vi "INI Use Position Size.vi"(8 "error in":errorcluster, 11 "Editor Position in":refnum<class "Editor Position.lvclass">) -> (0 "error out":errorcluster, 3 "Editor Position out":refnum<class "Editor Position.lvclass">)   [LabVIEW 2021, in "Editor Position.lvclass"]
doc: "Tests the reading of the Use Position Size INI key."
uses:
  Editor Position.lvclass
  C:/Program Files/National Instruments/LabVIEW 2024/vi.lib/Astemes/LUnit/Test Case.lvclass
  <vilib>/Astemes/LUnit/Test Case.lvclass/Test Case.ctl
  <vilib>/Astemes/LUnit/Core/LUnit Test Case/Private/Append Pass Result.vi
  <vilib>/Astemes/LUnit/Core/LUnit Test Case/Private/Append Fail Result.vi
  <vilib>/Astemes/LUnit/Core/LUnit Test Case/Private/Run In UI.vi
  <vilib>/Utility/error.llb/Clear Errors.vi
  <resource>/dialog/lvconfig.llb/LV Config Write Boolean.vi
  <vilib>/LabVIEW Icon API/lv_icon/lv_icon.lvlib
  <vilib>/Astemes/LUnit/Test Case.lvclass
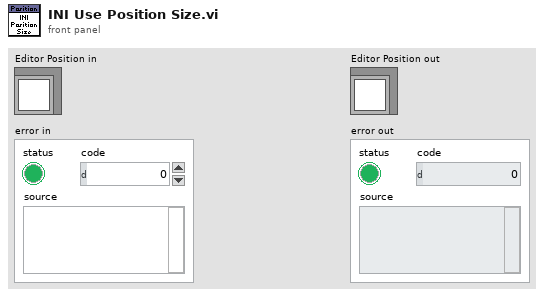
[diagram p1: front panel]
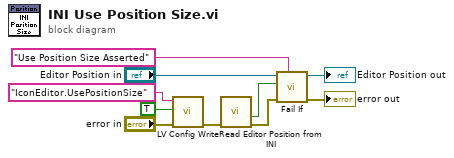
[diagram p0: block diagram]
diagram:
  n1 = call-poly <resource>:"LV Config Write.vi"("error in (no error)"="error in", "value"=TRUE, "key"="IconEditor.UsePositionSize") -> ("error out"=w7:errorcluster)  [unwired: 4 in]
  n2 = call <resource>:"Read Editor Position from INI.vi"("error in"=w7) -> ("error out"=w10:errorcluster, "Use Size"=w4:bool)  [unwired: 7 in, 2 out]
  n3 = call <vilib>:"Fail If.vi"("Description"="Use Position Size Asserted", "error in (no error)"=w10, "Fail?"=w4, "LUnit Test Case In"="Editor Position in") -> ("error out"=→"error out":errorcluster, "LUnit Test Case Out"=→"Editor Position out":refnum<class "Editor Position.lvclass">)  [unwired: 6 in]
